vi "exersise 3-2.vi"() -> ()   [LabVIEW 2014]
panel:
  out "number of iterations":i32
  out "final random number":dbl
  in  "number between 0 and 1000":dbl
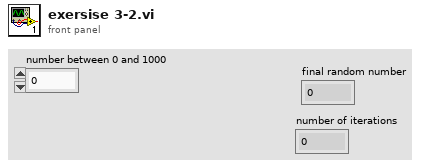
[diagram p1: front panel]
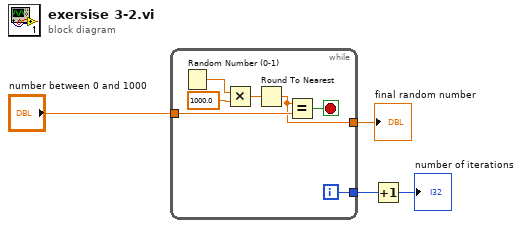
[diagram p0: block diagram]
diagram:
  n1 = while {
    tunnel: [w11] -> w2
    tunnel: "number between 0 and 1000" -> [w8]
    tunnel: [w5] -> w3
    i -> [w11]
    stop <- w7 stop-if-true
    n2 = Random Number (0-1)() -> (number: 0 to 1=w10:dbl)
    n3 = Multiply(x=w10, y=1000.0) -> (x*y=w6:dbl)
    n4 = Round To Nearest(number=w6) -> (nearest integer value=w5:dbl)
    n5 = Equal?(x=w5, y=w8) -> (x = y?=w7:bool)
  }
  "final random number" <- w3
  n6 = Increment(x=w2) -> (x+1=→"number of iterations":i32)
